vi "finishTableWithStrikerPlay.vi"(10 "Game":refnum<class "Game.lvclass">, 11 "TableWithStrikerPlay in":refnum<class "TableWithStrikerPlay.lvclass">) -> (2 "finishTableWith2ndStriker?":bool, 3 "TableWithStrikerPlay out":refnum<class "TableWithStrikerPlay.lvclass">)   [LabVIEW 2020, in "TableWithStrikerPlay.lvclass"]
uses:
  TableWithStrikerPlay.lvclass
  Game_class/Game.lvclass
  C:/Users/Administrator/Desktop/SSL/SSL_AI/Play_class/Play.lvclass
  Referee_class/command_interpreted.ctl
  Game_class/Game.lvclass/Game.ctl
  Referee_class/Referee.lvclass/Referee.ctl
  Events_class/Events.lvclass/Events.ctl
  Ball_class/Ball.lvclass/Ball.ctl
  Team_class/Team.lvclass/Team.ctl
  Game_class/Read EventsRef.vi
  Game_class/Read BallRef.vi
  Game_class/Read OffensiveTeam.vi
  Team_class/Read RobotRef.vi
  Ball_class/Read z.vi
  Events_class/Read touch.vi
  Events_class/Read id_touch.vi
  Events_class/Read ball_out.vi
  Game_class/Read Referee.vi
  Referee_class/Read command_interpreted.vi
  Ally_class/Ally.lvclass
  C:/Users/Administrator/Desktop/SSL/SSL_AI/Team_class/Team.lvclass
  Referee_class/Referee.lvclass
  Events_class/Events.lvclass
  Ball_class/Ball.lvclass
  Robot_class/Robot.lvclass
  Play_class/Play.lvclass
panel:
  out "error out":errorcluster
  in  "error in (no error)":errorcluster
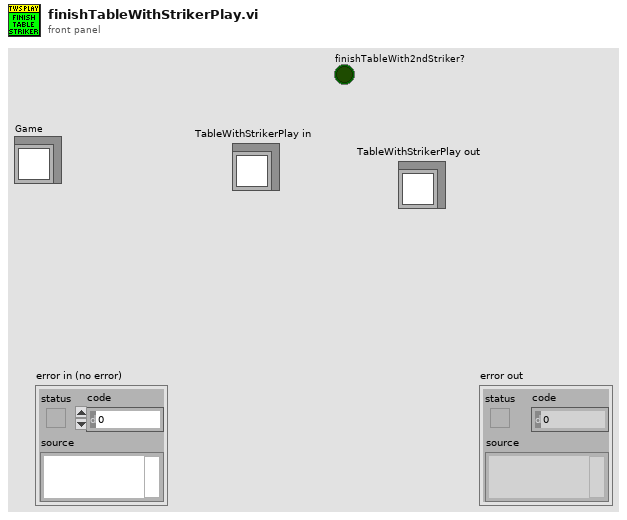
[diagram p1: front panel]
types:
  T1 = typedef "command_interpreted.ctl" = enum16{"Goal Ally", "Goal Enemy", "Ball Placement Enemy", "Ball Placement Ally", "Normal Half Time", "Extra Time  Break", "Extra Half Time", "None", "Post Game", "PKA Normal Start", "Prepare Kickoff Ally", "PKE Normal Start", "Prepare Kickoff Enemy", "Force Start", "Halt", "Timeout", "Prepare Penalty Ally", "Prepare Penalty Enemy", "PPA NormalStart", "PPE Normal Start", "Indirect Free Ally", "Direct Free Enemy", "Direct Free Ally", "Indirect Free Enemy", "Stop"}
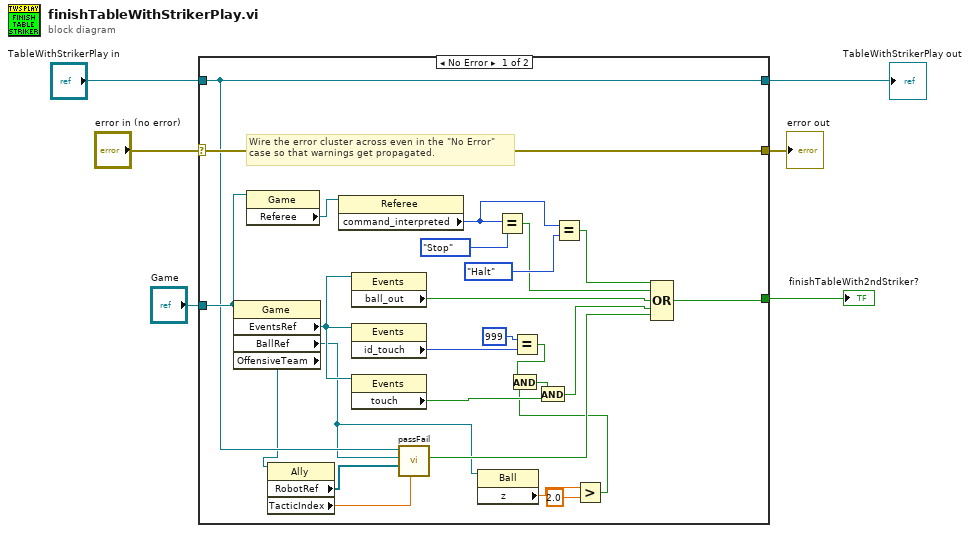
[diagram p0: block diagram]
diagram:
  n1 = case shown="No Error" "error in (no error)" {
    selector: "error in (no error)" -> [w32 w34]
    tunnel: [w32 w34] -> w5
    tunnel: [w22 w33] -> w1
    tunnel: "TableWithStrikerPlay in" -> [w22 w33]
    tunnel: [w18 _] -> w4
    tunnel: "Game" -> [w26 _]
    frame No Error {
      # "Wire the error cluster across even in the \"No Error\"\ncase so that warnings get propagated."
      n2 = property class="Game"(reference=w26) -> ("EventsRef"=w31:refnum<class "Events.lvclass">, "BallRef"=w10:refnum<class "Ball.lvclass">, "OffensiveTeam"=w21:refnum<class "Ally.lvclass">)  [unwired: 1 in, 2 out]
      n3 = property class="Game"(reference=w26) -> ("Referee"=w28:refnum<class "Referee.lvclass">)  [unwired: 1 in, 2 out]
      n4 = property class="Ally"(reference=w21) -> ("RobotRef"=w20:refnum<class "Robot.lvclass">[], "TacticIndex"=w19:dbl)  [unwired: 1 in, 2 out]
      n5 = property class="Referee"(reference=w28) -> ("command_interpreted"=w24:T1)  [unwired: 1 in, 2 out]
      n6 = property class="Events"(reference=w31) -> ("ball_out"=w15:bool)  [unwired: 1 in, 2 out]
      n7 = property class="Events"(reference=w31) -> ("id_touch"=w29:i32)  [unwired: 1 in, 2 out]
      n8 = property class="Events"(reference=w31) -> ("touch"=w27:bool)  [unwired: 1 in, 2 out]
      n9 = call "passFail.vi"("TacticIndex"=w19, "Offensive Robots"=w20, "Ball"=w10, "Play in"=w22) -> ("PassFail?"=w13:bool)  [unwired: 5 in, 2 out]
      n10 = property class="Ball"(reference=w10) -> ("z"=w12:dbl)  [unwired: 1 in, 2 out]
      n11 = Equal?(x=w24, y=command_interpreted."Stop") -> (x = y?=w16:bool)
      n12 = Equal?(x=999 ("id_touch"), y=w29) -> (x = y?=w8:bool)
      n13 = Equal?(x=w24, y=command_interpreted."Halt") -> (x = y?=w17:bool)
      n14 = Greater?(x=w12, y=2.0) -> (0:w9:bool)
      n15 = And(x=w8, y=w9) -> (x .and. y?=w7:bool)
      n16 = And(x=w7, y=w27) -> (x .and. y?=w14:bool)
      n17 = Compound Arithmetic op=OR(w17, w16, w15, w14, w13) -> (w18:bool)
    }
    frame Error {
    }
  }
  "error out" <- w5
  "finishTableWith2ndStriker?" <- w4
  "TableWithStrikerPlay out" <- w1
